vi "_RT_CtrlLoop_Safty.vi"(6 "system state":refnum<data-value>, 8 "error in (no error)":errorcluster, 10 "safty":refnum<data-value>, 11 "system enable":refnum<data-value>) -> ()   [LabVIEW 2018]
uses:
  PublicSubVI/Ctl/_ctl_RT_System_State.ctl
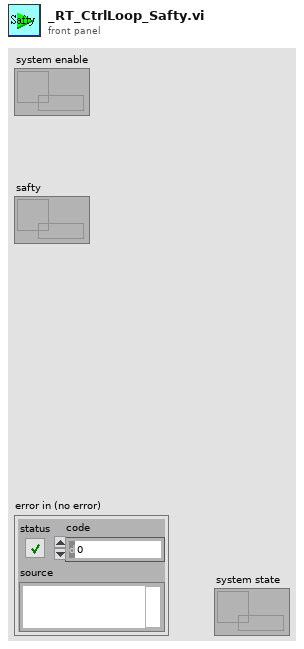
[diagram p1: front panel]
types:
  T1 = typedef "_ctl_RT_System_State.ctl" = enum16{"initialize", "idle", "working", "disconnect"}
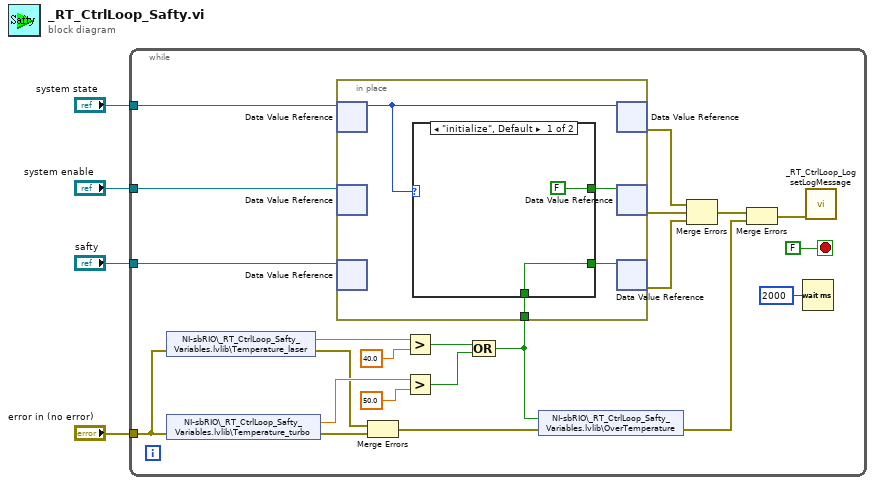
[diagram p0: block diagram]
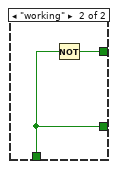
[diagram p2: hidden frame]
diagram:
  n1 = while {
    tunnel: "error in (no error)" -> [w21]
    tunnel: "system enable" -> [w18]
    tunnel: "system state" -> [w14]
    tunnel: "safty" -> [w15]
    stop <- FALSE stop-if-true
    n2 = shared-variable "NI-sbRIO\\_RT_CtrlLoop_Safty_Variables.lvlib\\Temperature_laser"(error in=w21) -> (w25:sgl, error out=w20:errorcluster)
    n3 = shared-variable "NI-sbRIO\\_RT_CtrlLoop_Safty_Variables.lvlib\\Temperature_turbo"(error in=w21) -> (w24:sgl, error out=w19:errorcluster)
    n4 = Merge Errors(w20, w19) -> (w8:errorcluster)
    n5 = Greater?(x=w25, y=sgl 40.0) -> (0:w17:bool)
    n6 = Greater?(x=w24, y=sgl 50.0) -> (0:w22:bool)
    n7 = Compound Arithmetic op=OR(w17, w22) -> (w16:bool)
    n8 = in-place {
      in-place-border: w16 -> [w29]
      n9 = in-place-dvr #1(w14) -> (w27:T1)  [unwired: 1 out]
      n10 = in-place-dvr #2(w18) -> ()  [unwired: 2 out]
      n11 = in-place-dvr #3(w15) -> ()  [unwired: 2 out]
      n12 = case shown="\"initialize\", Default" w27 {
        tunnel: [FALSE w34] -> w30
        tunnel: w29 -> [w32 w33]
        tunnel: [w32 w33] -> w28
        frame "initialize", Default {
        }
        frame "working" {
          n13 = Not(x=w33) -> (.not. x?=w34:bool)
        }
      }
      n14 = in-place-dvr #1(w27) -> (w12:errorcluster)  [unwired: 1 out]
      n15 = in-place-dvr #2(w30) -> (w13:errorcluster)  [unwired: 1 out]
      n16 = in-place-dvr #3(w28) -> (w11:errorcluster)  [unwired: 1 out]
    }
    n17 = shared-variable "NI-sbRIO\\_RT_CtrlLoop_Safty_Variables.lvlib\\OverTemperature"(w16, error in=w8) -> (error out=w7:errorcluster)
    n18 = Merge Errors(w12, w13, w11) -> (w10:errorcluster)
    n19 = Merge Errors(w10, w7) -> (w9:errorcluster)
    n20 = Wait (ms)(milliseconds to wait=u32 2000) -> ()  [unwired: 1 out]
    n21 = call "_RT_CtrlLoop_Log setLogMessage.vi"("error in"=w9) -> ()  [unwired: 9 in, 2 out]
  }
